vi "DaNIDemoVI.vi"() -> ()   [LabVIEW 2016]
uses:
  <vilib>/userdefined/High Color/nirio_resource_hc.ctl
  <vilib>/Analysis/Matrix/Numeric/Conversions/Array To Matrix - RA.vi
  <vilib>/Analysis/Matrix/Numeric/Multiply/Multiply - RM,RM.vi
  <vilib>/Analysis/Matrix/Numeric/Subtract/Subtract - RM,RM.vi
  <vilib>/Analysis/Matrix/NI_Matrix.lvlib
panel:
  in  "B _L":dbl[](array[numeric])
  in  "A _L":dbl[](array[numeric])
  in  "B _R":dbl[](array[numeric])
  in  "A _R":dbl[](array[numeric])
  out "current setpoint":dbl
  in  "lamda":i32
  in  "Horizon":i32
  out "Waveform Chart 2":dbl(graph)
  out "Waveform Chart":dbl(graph)
  in  "Mode Select":T1(ring)
  in  "IP Adress":T2="rio://169.254.0.1/RIO0"
  out "Distance Measured (m)":dbl
  in  "Servomotor Angle Offset (Degrees)":dbl
  in  "Servomotor Angle (Degrees)":dbl
  out "Rad/s Right":dbl
  out "Rad/s Left":dbl
  in  "dt (ms)":u32=50
  out "Right Motor Voltage Percentage In (-1 to 1)":dbl min=-1.0 max=1.0 step=0.01
  out "Left Motor Voltage Percentage In (-1 to 1)":dbl min=-1.0 max=1.0 step=0.01
  in  "stop":bool
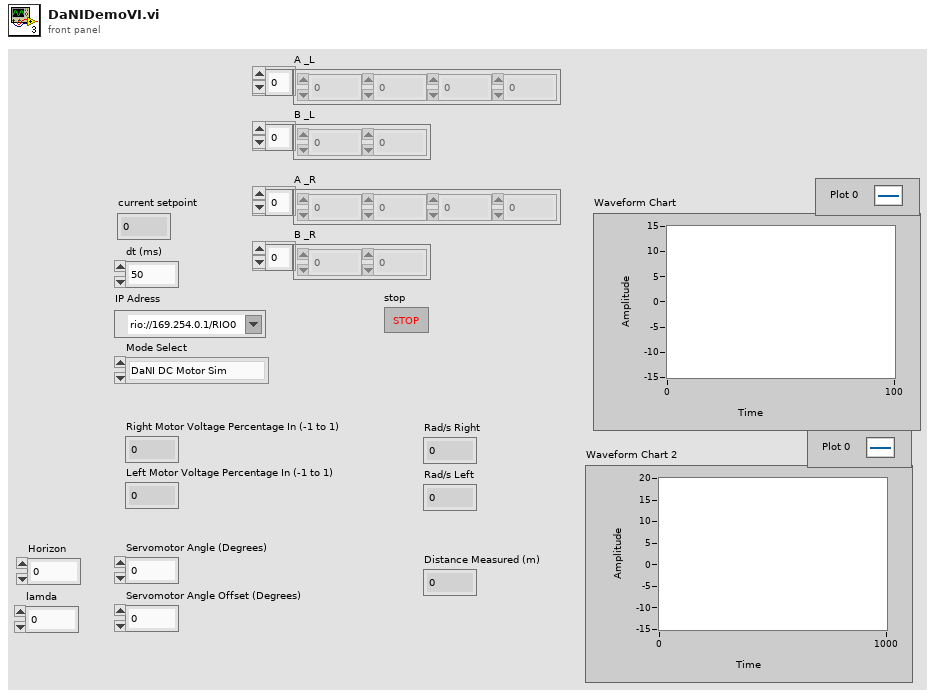
[diagram p1: front panel]
types:
  T1 = enum16{"DaNI DC Motor Sim", "DaNI Simulation", "DaNI Robot"}
  T2 = typedef "nirio_resource_hc.ctl" = tag
  T3 = typedef "NI_Matrix.lvlib/RealMatrix.ctl" = dbl[][]
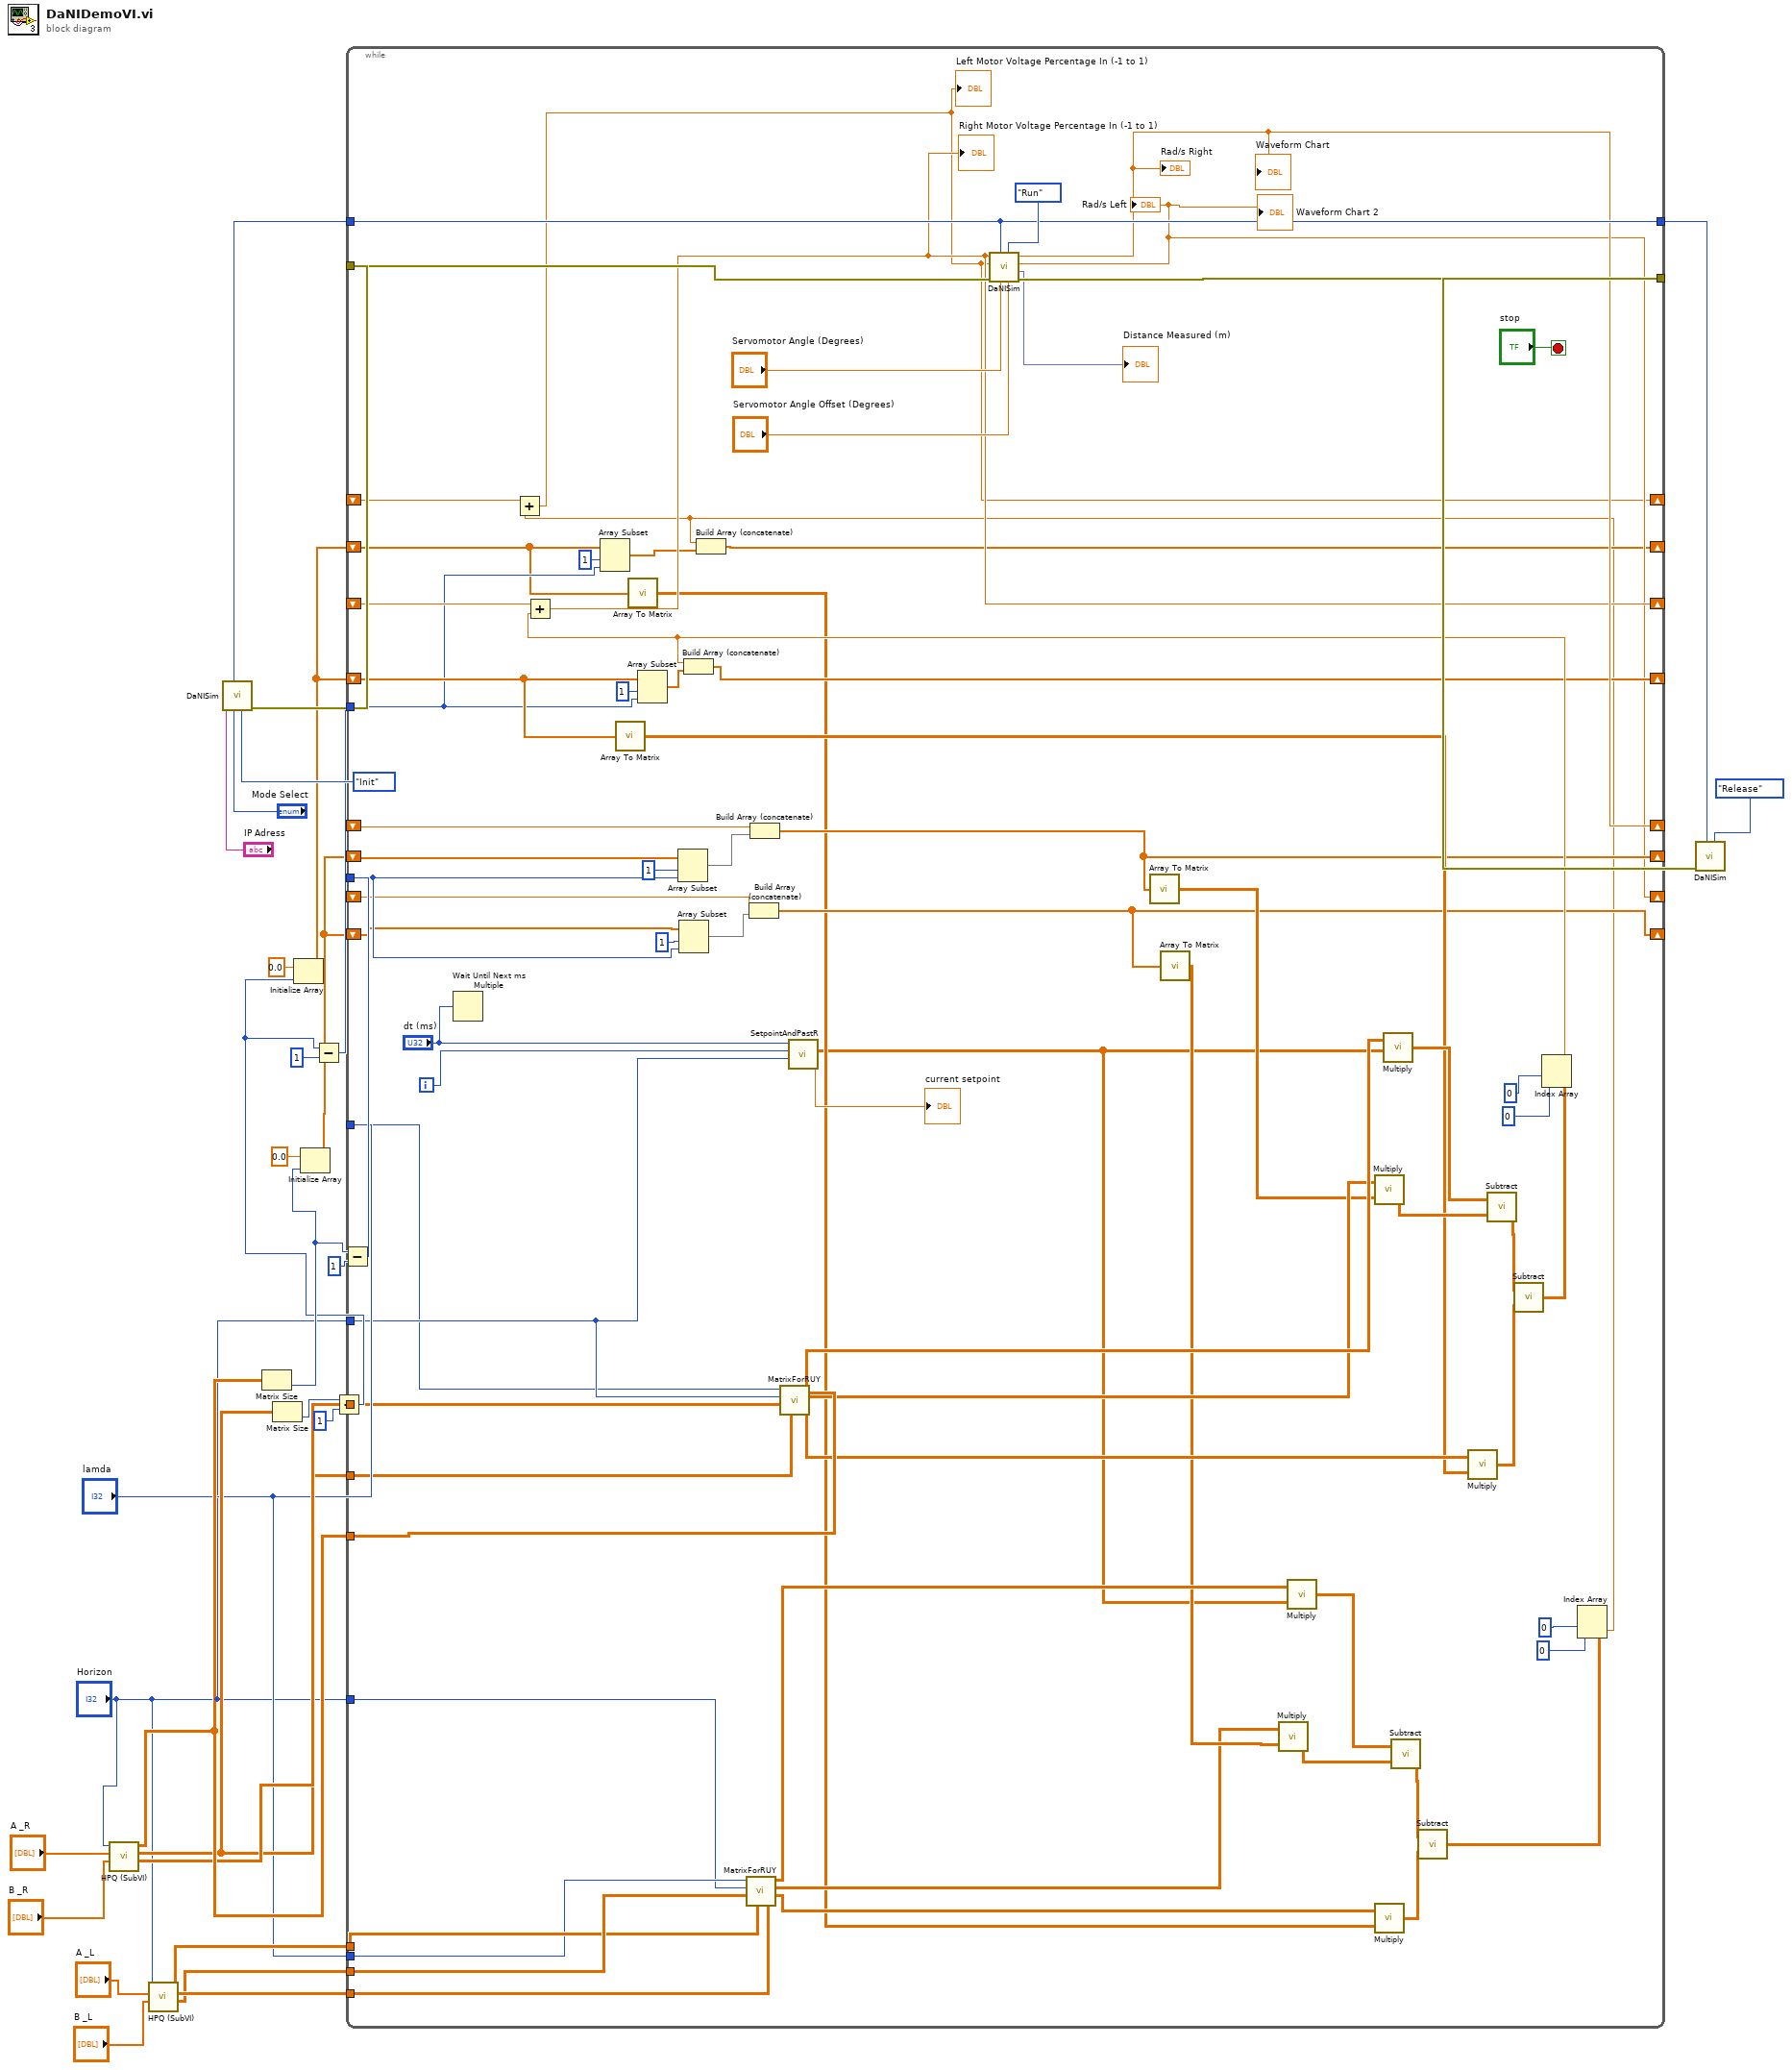
[diagram p0: block diagram]
diagram:
  n1 = call "HPQ (SubVI).vi"("B"="B _R", "A"="A _R", "Horizon"="Horizon") -> ("H"=w11:T3, "P"=w10:T3, "Q"=w12:T3)  [unwired: 6 in]
  n2 = call "HPQ (SubVI).vi"("B"="B _L", "A"="A _L", "Horizon"="Horizon") -> ("H"=w6:T3, "P"=w7:T3, "Q"=w5:T3)  [unwired: 6 in]
  n3 = call "DaNISim.vi"("Action"=enum16{"Init", "Run", "Release"}."Init", "Mode Select"="Mode Select", "IP Adress"="IP Adress") -> ("error out"=w29:errorcluster)  [unwired: 5 in, 3 out]
  n4 = Matrix Size(0:w12) -> (2:w19:i32)  [unwired: 1 out]
  n5 = Matrix Size(0:w10) -> (2:w22:i32)  [unwired: 1 out]
  n6 = Initialize Array(0.0 ("element"), w19) -> (w1:dbl[])
  n7 = Subtract(x=w22, y=1) -> (x-y=w17:i32)
  n8 = Initialize Array(0.0 ("element"), w17) -> (w2:dbl[])
  n9 = Subtract(x=w17, y=1) -> (x-y=w15:i32)
  n10 = Subtract(x=w19, y=1) -> (x-y=w18:i32)
  n11 = while {
    tunnel: w29 -> [w104]
    tunnel: "Mode Select" -> [w98]
    tunnel: [w102] -> w27
    tunnel: [w98] -> w25
    shift-right: [w94] -> _
    shift-left: _ -> [w87]
    tunnel: w12 -> [w93]
    tunnel: w10 -> [w92]
    tunnel: w11 -> [w91]
    tunnel: "Horizon" -> [w90]
    tunnel: "lamda" -> [w89]
    shift-right: [w61] -> _
    shift-left: w1 -> [w86]
    shift-right: [w67] -> _
    shift-left: _ -> [w76]
    shift-right: [w72] -> _
    shift-left: w2 -> [w70]
    tunnel: w18 -> [w59]
    tunnel: w15 -> [w52]
    tunnel: w7 -> [w66]
    tunnel: w6 -> [w65]
    tunnel: w5 -> [w64]
    tunnel: "lamda" -> [w63]
    tunnel: "Horizon" -> [w62]
    shift-right: [w57] -> _
    shift-left: _ -> [w33]
    shift-right: [w55] -> _
    shift-left: w1 -> [w56]
    shift-right: [w49] -> _
    shift-left: _ -> [w54]
    shift-right: [w50] -> _
    shift-left: w2 -> [w48]
    i -> [w97]
    stop <- "stop" stop-if-true
    n12 = Wait Until Next ms Multiple(millisecond multiple="dt (ms)") -> ()  [unwired: 1 out]
    n13 = Array Subset(array=w48, index=1, length=w52) -> (w51:dbl[])
    n14 = call-poly <vilib>:"Array To Matrix.vi"("Real 1D Array"=w70) -> ("Real Matrix (Column Vector)"=w69:T3)
    n15 = call-poly <vilib>:"Array To Matrix.vi"("Real 1D Array"=w48) -> ("Real Matrix (Column Vector)"=w35:T3)
    n16 = Array Subset(array=w70, index=1, length=w52) -> (w74:dbl[])
    n17 = Array Subset(array=w86, index=1, length=w59) -> (w88:dbl[])
    n18 = Array Subset(array=w56, index=1, length=w59) -> (w58:dbl[])
    n19 = call "MatrixForRUY.vi"("P"=w66, "Q"=w64, "H"=w65, "Horizon"=w62, "lamda"=w63) -> ("M_U"=w40:T3, "M_Y"=w36:T3, "M_R"=w39:T3)  [unwired: 4 in]
    n20 = Build Array (concatenate)(w33, w58) -> (w55:dbl[])
    n21 = Build Array (concatenate)(w87, w88) -> (w61:dbl[])
    n22 = call "MatrixForRUY.vi"("P"=w92, "Q"=w93, "H"=w91, "Horizon"=w90, "lamda"=w89) -> ("M_U"=w71:T3, "M_Y"=w84:T3, "M_R"=w95:T3)  [unwired: 4 in]
    n23 = call "SetpointAndPastR.vi"("Horizon"=w90, "i"=w97, "dt (ms)"="dt (ms)") -> ("Future_R"=w32:T3, "b"=→"current setpoint":dbl)  [unwired: 7 in]
    n24 = call-poly <vilib>:"Array To Matrix.vi"("Real 1D Array"=w61) -> ("Real Matrix (Column Vector)"=w83:T3)
    n25 = call-poly <vilib>:"Array To Matrix.vi"("Real 1D Array"=w55) -> ("Real Matrix (Column Vector)"=w37:T3)
    n26 = call-poly <vilib>:"Multiply.vi"("Real Matrix B"=w37, "Real Matrix A"=w36) -> ("A * B"=w46:T3)
    n27 = call-poly <vilib>:"Multiply.vi"("Real Matrix B"=w32, "Real Matrix A"=w39) -> ("A * B"=w47:T3)
    n28 = call-poly <vilib>:"Multiply.vi"("Real Matrix B"=w83, "Real Matrix A"=w84) -> ("A * B"=w81:T3)
    n29 = call-poly <vilib>:"Multiply.vi"("Real Matrix B"=w35, "Real Matrix A"=w40) -> ("A * B"=w41:T3)
    n30 = call-poly <vilib>:"Multiply.vi"("Real Matrix B"=w32, "Real Matrix A"=w95) -> ("A * B"=w82:T3)
    n31 = call-poly <vilib>:"Subtract.vi"("Real Matrix B"=w46, "Real Matrix A"=w47) -> ("A - B"=w45:T3)
    n32 = call-poly <vilib>:"Subtract.vi"("Real Matrix B"=w41, "Real Matrix A"=w45) -> ("A - B"=w44:T3)
    n33 = call-poly <vilib>:"Multiply.vi"("Real Matrix B"=w69, "Real Matrix A"=w71) -> ("A * B"=w68:T3)
    n34 = call-poly <vilib>:"Subtract.vi"("Real Matrix B"=w81, "Real Matrix A"=w82) -> ("A - B"=w80:T3)
    n35 = call-poly <vilib>:"Subtract.vi"("Real Matrix B"=w68, "Real Matrix A"=w80) -> ("A - B"=w79:T3)
    n36 = Index Array(array=w79, index (row)=0 ("disabled index (row)"), index (col)=0 ("disabled index (col)")) -> (element=w73:dbl)
    n37 = Add(x=w76, y=w73) -> (x+y=w67:dbl)
    "Right Motor Voltage Percentage In (-1 to 1)" <- w67
    n38 = Build Array (concatenate)(w73, w74) -> (w72:dbl[])
    n39 = Index Array(array=w44, index (row)=0 ("disabled index (row)"), index (col)=0 ("disabled index (col)")) -> (element=w34:dbl)
    n40 = Add(x=w54, y=w34) -> (x+y=w49:dbl)
    "Left Motor Voltage Percentage In (-1 to 1)" <- w49
    n41 = Build Array (concatenate)(w34, w51) -> (w50:dbl[])
    n42 = call "DaNISim.vi"("Sonar offset angle"="Servomotor Angle Offset (Degrees)", "Action"=enum16{"Init", "Run", "Release"}."Run", "Sonar angle"="Servomotor Angle (Degrees)", "Mode Select"=w98, "error in (no error)"=w104, "Ul"=w49, "Ur"=w67) -> ("error out"=w102:errorcluster, "Sonar distance"=→"Distance Measured (m)":fxp<+,32,8>, "OmegaL"=w57:dbl, "OmegaR"=w94:dbl)  [unwired: 1 in]
    "Rad/s Left" <- w57
    "Rad/s Right" <- w94
    "Waveform Chart" <- w94
    "Waveform Chart 2" <- w57
  }
  n43 = call "DaNISim.vi"("Action"=enum16{"Init", "Run", "Release"}."Release", "Mode Select"=w25, "error in (no error)"=w27) -> ()  [unwired: 5 in, 4 out]
